vi "Config Hyperion.vi"() -> ()   [LabVIEW 2016]
uses:
  hyperion library source/h.Library/DETECTION/h.DETECTION.PeakDetectionPreset.ctl
  hyperion library source/h.Library.lvlib
panel:
  out "Instrument Detection Settings":T1[](array[typedef])
  in  "Detection Setting 2":T1={"Index"=0, "Name"="", "Description"="", "Detection Mode"=enum."Peak", "Averaging Window (pm)"=0, "Peak Width (pm)"=1000, "Lockout Period (pm)"=0, "Search Window (ps)"=0, "Threshold Level"=0}
  in  "Detection Setting Index":u8
  out "Detection Setting":T1
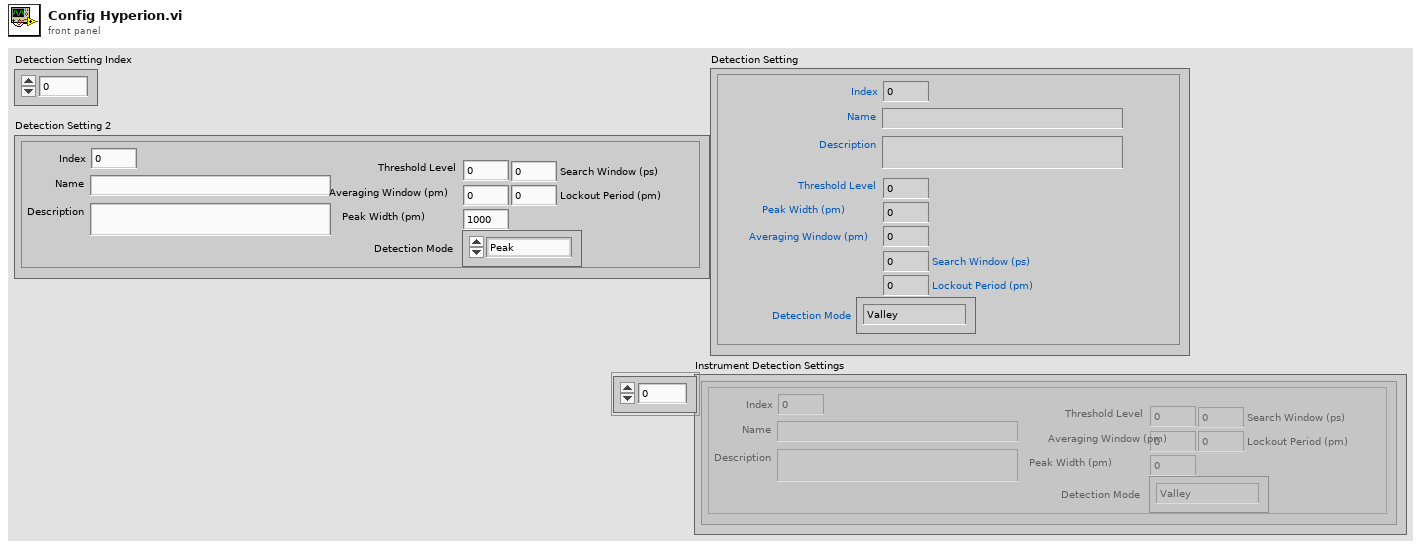
[diagram p1: front panel]
types:
  T1 = typedef "h.Library.lvlib/h.DETECTION.PeakDetectionPreset.ctl" = cluster{"Index":u8, "Name":string, "Description":string, "Detection Mode":enum32{"Valley", "Peak"}, "Averaging Window (pm)":i32, "Peak Width (pm)":i32, "Lockout Period (pm)":i32, "Search Window (ps)":i32, "Threshold Level":i32}
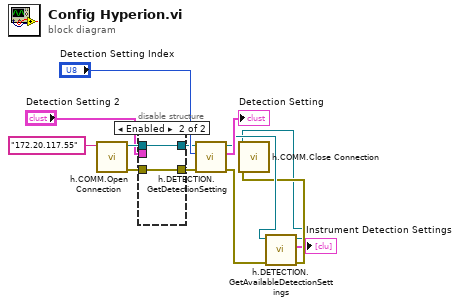
[diagram p0: block diagram]
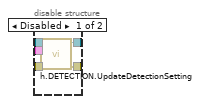
[diagram p2: hidden frame]
diagram:
  n1 = call "h.COMM.Open Connection.vi"("Address"="172.20.117.55") -> ("error out"=w9:errorcluster, "Connection ID"=w10:refnum<k5>)  [unwired: 9 in]
  n2 = disable-structure shown="Enabled" {
    disable-tunnel: w10 -> [w18 w20]
    disable-tunnel: w9 -> [w17 w19]
    disable-tunnel: [w16 w19] -> w8
    disable-tunnel: [w15 w20] -> w7
    disable-tunnel: "Detection Setting 2" -> [w14 _]
    frame Disabled {
      n3 = call "h.DETECTION.UpdateDetectionSetting.vi"("error in"=w17, "Detection Setting"=w14, "Connection ID"=w18) -> ("error out"=w16:errorcluster, "Connection ID out"=w15:refnum<k5>)  [unwired: 7 in]
    }
    frame Enabled {
    }
  }
  n4 = call "h.DETECTION.GetDetectionSetting.vi"("error in"=w8, "Detection Setting Index"="Detection Setting Index", "Connection ID"=w7) -> ("error out"=w4:errorcluster, "Detection Setting"=→"Detection Setting":T1, "Connection ID out"=w5:refnum<k5>)  [unwired: 6 in]
  n5 = call "h.DETECTION.GetAvailableDetectionSettings.vi"("error in"=w4, "Connection ID"=w5) -> ("error out"=w3:errorcluster, "Instrument Detection Settings"=→"Instrument Detection Settings":T1[], "Connection ID out"=w2:refnum<k5>)  [unwired: 7 in]
  n6 = call "h.COMM.Close Connection.vi"("error in"=w3, "Connection ID"=w2) -> ()  [unwired: 9 in, 1 out]
